vi "UDP Remote IP to String Test.vi"() -> ()   [LabVIEW 2014, in "ESP8266 WiFi Wrapper.lvlib"]
uses:
  <vilib>/Aledyne-TSXperts/Arduino Compatible Compiler for LabVIEW/addons/ESP8266 WiFi Wrapper/ESP8266 WiFi Wrapper.lvlib
panel:
  out "Remote IP":string
  out "Error Out":errorcluster
  in  "Error In":errorcluster
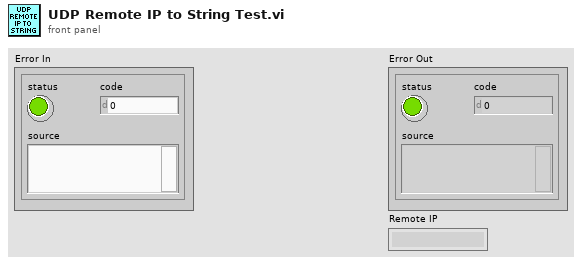
[diagram p1: front panel]
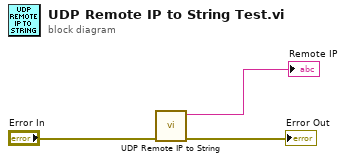
[diagram p0: block diagram]
diagram:
  n1 = call <vilib>:"UDP Remote IP to String.vi"("Error In"="Error In") -> ("Error Out"=→"Error Out":errorcluster, "Remote IP"=→"Remote IP":string)  [unwired: 9 in]
